vi "Test Compare Equal Nested Clusters.vi"(11 "Compare Assertion Test In":refnum<class "Compare Assertion Test.lvclass">) -> (0 "error out":errorcluster, 3 "Compare Assertion Test Out":refnum<class "Compare Assertion Test.lvclass">)   [LabVIEW 2020, in "Compare Assertion Test.lvclass"]
uses:
  Compare Assertion Test.lvclass
  C:/Program Files (x86)/National Instruments/LabVIEW 2020/vi.lib/Astemes/LUnit/Test Case.lvclass
  Comparison Test Double/Test Methods.ctl
  source/Core/Result/Status.ctl
  <vilib>/Astemes/LUnit/Test Case.lvclass/Test Case.ctl
  e8fb4b8a-135a-4145-a117-571442495440.vi
  <vilib>/Astemes/LUnit/Append Pass Result.vi
  <vilib>/Astemes/LUnit/Append Fail Result.vi
  <vilib>/Astemes/LUnit/Describe Comparison.vi
  e8fb4b8a-135a-4145-a117-571442495440.vi/9c5d11cd-9439-4240-a1ee-d9baace9c924.vi
  <vilib>/Astemes/LUnit/Run In UI.vi
  <vilib>/Utility/error.llb/Clear Errors.vi
  <vilib>/Astemes/LUnit/Describe Variant.vi
  Compare Assertion Test.lvclass/Compare Assertion Test.ctl
  Comparison Test Double/Comparison Test Double.lvclass
  source/Core/Result/Result.lvlib
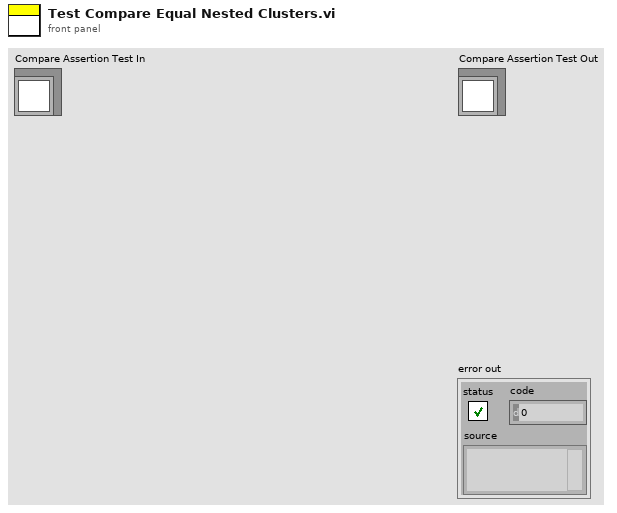
[diagram p1: front panel]
types:
  T1 = typedef "Result.lvlib/Status.ctl" = enum16{"", "Passed", "Failed", "Error", "Skipped", "Setup Error", "Broken", "Teardown Error"}
  T2 = typedef "Comparison Test Double.lvclass/Test Methods.ctl" = enum16{"Test Compare Equal Enums.vi", "Test Compare Unequal Enums.vi", "Test Compare Equal Strings.vi", "Test Compare Unequal Type Deffed Enums.vi", "Test Compare Equal 8bit Enums.vi", "Test Compare Equal 1el String Arrays.vi", "Test Compare Fail if Equal 1el String Arrays.vi", "Test Compare Array with Tolerance.vi", "Test Compare Equal Strings one as Variant.vi", "Test Compare Equal Strings Other as Variant.vi", "Test Compare Equal Variants.vi", "Test Compare Equal Clusters.vi", "Test Compare Equal Nested Clusters.vi"}
  T3 = typedef "Result.lvlib/Result.ctl" = cluster{"Name":string, "Message":string, "Description":string, "Status":T1, "Result Type":T4, "Execution Time":dbl}
  T4 = typedef "Result.lvlib/Type.ctl" = enum16{"Test Case", "Test Suite", "Test Run", "Pass", "Fail", "Skip", "Pass if", "Fail if", "Pass if Error", "Fail if Error", "Pass if Equal", "Fail if Equal"}
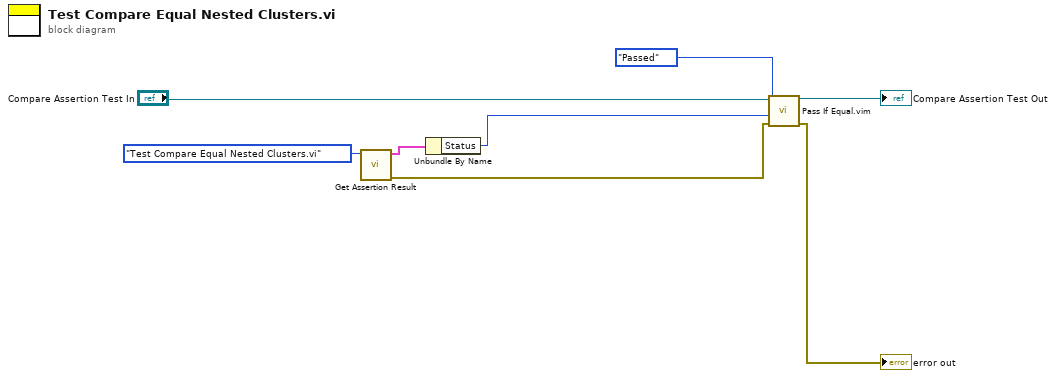
[diagram p0: block diagram]
diagram:
  n1 = call "Get Assertion Result.vi"("Test VIs"=Test_Methods."Test Compare Equal Nested Clusters.vi") -> ("error out"=w1:errorcluster, "First Result"=w4:T3)  [unwired: 8 in, 1 out]
  n2 = Unbundle By Name(w4) -> ("Status"=w3:T1)
  n3 = call "Pass If Equal.vim"("error in (no error)"=w1, "Actual"=w3, "Expected"=Status."Passed" ("Status"), "LUnit Test Case In"="Compare Assertion Test In") -> ("error out"=→"error out":errorcluster, "LUnit Test Case Out"=→"Compare Assertion Test Out":refnum<class "Compare Assertion Test.lvclass">)  [unwired: 6 in]
